vi "Komponente nicht mehr mit selber Formel.vi"(10 "neue Komponente":u16, 11 "alte Kompomente":u16) -> (3 "geändert":bool)   [LabVIEW 2020, in "EPA 1065.lvlib" / "HovaCAL Interference verificaton.lvlib"]
uses:
  HovaCAL Interference verificaton.lvlib
  Linearisierung V2/Gasteiler/Gasteiler.lvlib
  Linearisierung V2/Gasteiler/Aktion FGV Gasteilerliste laden.ctl
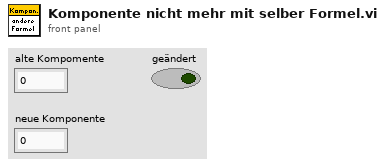
[diagram p1: front panel]
types:
  T1 = typedef "Linearisierung v2.lvlib/Gasteiler.lvlib/Aktion FGV Gasteilerliste laden.ctl" = enum16{"lesen", "laden", "speichern", "Liste erstellen", "Formel ändern", "Gas vereinzeln"}
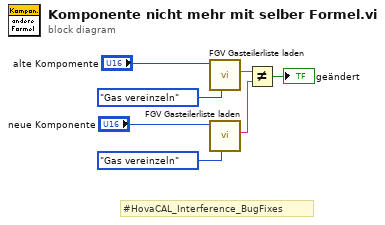
[diagram p0: block diagram]
diagram:
  # "#HovaCAL_Interference_BugFixes"
  n1 = call "FGV Gasteilerliste laden.vi"("Aktion"=Aktion_FGV_Gasteilerliste_laden."Gas vereinzeln", "Gasindex"="alte Kompomente") -> ("Formel"=w3:string)  [unwired: 7 in, 2 out]
  n2 = call "FGV Gasteilerliste laden.vi"("Aktion"=Aktion_FGV_Gasteilerliste_laden."Gas vereinzeln", "Gasindex"="neue Komponente") -> ("Formel"=w2:string)  [unwired: 7 in, 2 out]
  n3 = Not Equal?(x=w3, y=w2) -> (x != y?=→"geändert":bool)
